vi "波形数据属性与波形图绝对时间.vi"() -> ()   [LabVIEW 2012]
uses:
  <vilib>/measure/NI_MAPro.lvlib
panel:
  out "通道名=曲线名？":bool
  out "曲线.曲线名":string
  in  "X标尺.格式字符串":string="%<%H:%M\n%m:%d>T"
  out "波形图":waveform(dbl)(graph)
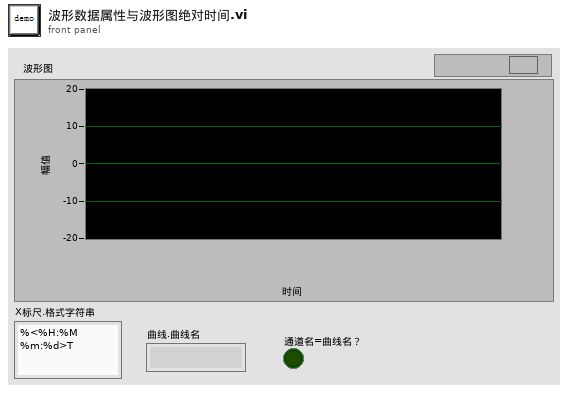
[diagram p1: front panel]
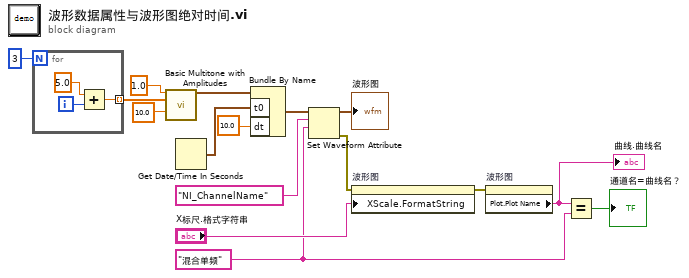
[diagram p0: block diagram]
diagram:
  w3 = "混合单频" ("名称")
  n1 = for {
    N: 3 -> [_]
    tunnel: [w17] -> w14 mode=indexing
    i -> [w19]
    n2 = Add(x=5.0, y=w19) -> (x+y=w17:dbl)
  }
  n3 = call <vilib>:"Basic Multitone with Amplitudes.vi"("start frequency"=1.0, "tone amplitudes"=w14, "delta frequency"=10.0) -> ("signal out"=w12:waveform(dbl))  [unwired: 9 in, 3 out]
  n4 = Get Date/Time In Seconds() -> (seconds since 1Jan1904=w11:timestamp)
  n5 = Bundle By Name(cluster=w12, "t0"=w11, "dt"=10.0) -> (w8:waveform(dbl))
  n6 = Set Waveform Attribute(5:w3, 6:"NI_ChannelName" ("名称"), 7:w8) -> (0:w4:errorcluster, 3:→"波形图":waveform(dbl))  [unwired: 1 in, 1 out]
  n7 = property on="波形图" class="WFGraph (严格)"(error in=w4, "XScale.FormatString"="X标尺.格式字符串") -> (error out=w5:errorcluster)  [unwired: 1 in, 1 out]
  n8 = property on="波形图" class="WFGraph (严格)"(error in=w5) -> ("Plot.Plot Name"=w2:string)  [unwired: 1 in, 2 out]
  "曲线.曲线名" <- w2
  n9 = Equal?(x=w2, y=w3) -> (x = y?=→"通道名=曲线名？":bool)
